vi "get_meas_env.vi"(10 "Stimuli":T3) -> (1 "Meas environment":T1, 2 "Load Set":T2)   [LabVIEW 2019]
doc: "Based on the stimuli cluster the VI generates the Load Set cluster and Meas environment cluster."
uses:
  ctl_stimuli_cluster.ctl
  ctl_loads_enum.ctl
  ctl_load_set_cluster.ctl
  ctl_meas_env_cluster.ctl
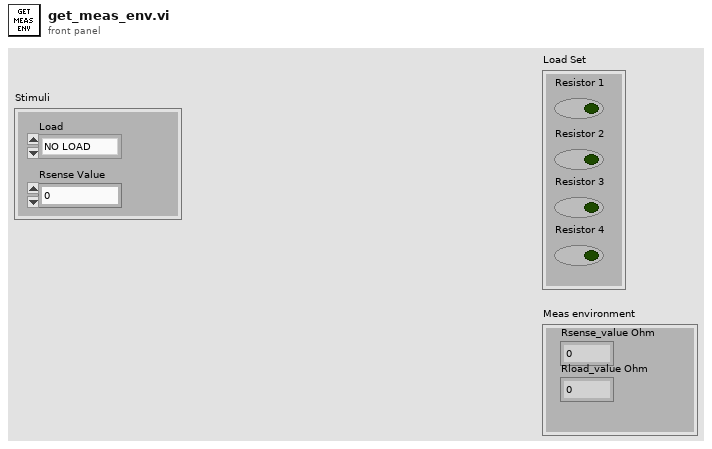
[diagram p1: front panel]
types:
  T1 = typedef "ctl_meas_env_cluster.ctl" = cluster{"Rsense_value Ohm":dbl, "Rload_value Ohm":dbl}
  T2 = typedef "ctl_load_set_cluster.ctl" = cluster{"Resistor 1":bool, "Resistor 2":bool, "Resistor 3":bool, "Resistor 4":bool}
  T3 = typedef "ctl_stimuli_cluster.ctl" = cluster{"Load":T4, "Rsense Value":dbl}
  T4 = typedef "ctl_loads_enum.ctl" = enum16{"NO LOAD"}
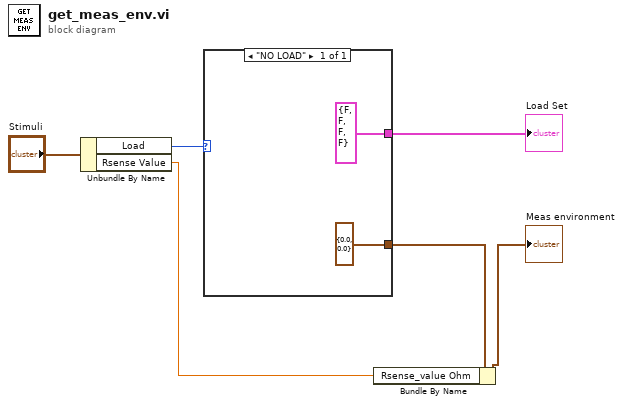
[diagram p0: block diagram]
diagram:
  n1 = Unbundle By Name("Stimuli") -> ("Load"=w4:T4, "Rsense Value"=w1:dbl)
  n2 = case shown="\"NO LOAD\"" w4 {
    tunnel: [T2 {"Resistor 1"=FALSE, "Resistor 2"=FALSE, "Resistor 3"=FALSE, "Resistor 4"=FALSE} ("Load Set")] -> w5
    tunnel: [T1 {"Rsense_value Ohm"=0.0, "Rload_value Ohm"=0.0} ("Meas environment")] -> w3
    frame "NO LOAD" {
    }
  }
  "Load Set" <- w5
  n3 = Bundle By Name(cluster=w3, "Rsense_value Ohm"=w1) -> (→"Meas environment":T1)
